vi "Lift Global.vi"() -> ()   [LabVIEW 2018]
panel:
  in  "Hatch Panel 1 Height":dbl
  out "Requested Height":dbl
  in  "Height PID":T1={"proportional gain (Kc)"=0.06, "integral time(Ti, min)"=0.0, "derivative time(Td, min) 2"=0.0}
  in  "Disable the VI":bool
  out "Current Lift Height":dbl
  in  "Cargo Zone 3 Height":dbl
  in  "Cargo Zone 2 Height":dbl
  in  "Cargo Zone 1 Height":dbl
  in  "Hatch Panel 3 Height":dbl
  in  "Hatch Panel 2 Height":dbl
  in  "CurrentState":T2(ring)
  out "Holding current position":bool
  out "Moving to position":bool
  in  "LiftHeight":dbl
  in  "Joystick manual":dbl
  in  "LiftMode":T3(ring)
  in  "LiftMotorSpeedDown":dbl
  in  "LiftLocation":T2(ring)
  in  "LiftMotorSpeedUp":dbl
  out "LowerLimit":bool=TRUE
  out "UpperLimit":bool
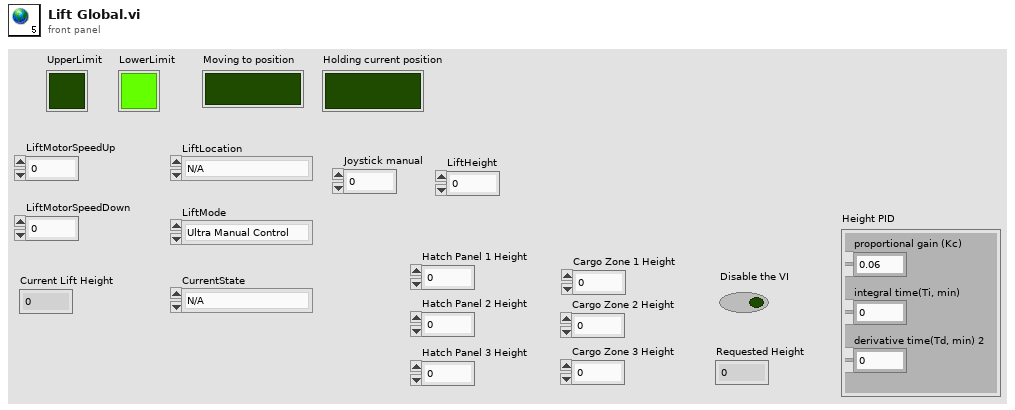
[diagram p1: front panel]
types:
  T1 = cluster{"proportional gain (Kc)":dbl, "integral time(Ti, min)":dbl, "derivative time(Td, min) 2":dbl}
  T2 = enum16{"N/A", "Hatch Panel Zone 1", "Hatch Panel Zone 2", "Hatch Panel Zone 3", "Cargo Zone 1", "Cargo Zone 2", "Cargo Zone 3"}
  T3 = enum16{"Ultra Manual Control", "Manual Control", "Basic Control", "Automated Control", "Autonomous Control"}
diagram:
